vi "Read presence_penalty.vi"(8 "error in (no error)":errorcluster, 11 "abstract_llm_base in":refnum<class "abstract_llm_base.lvclass">) -> (0 "error out":errorcluster, 2 "presence_penalty":dbl, 3 "abstract_llm_base out":refnum<class "abstract_llm_base.lvclass">)   [LabVIEW 2020, in "abstract_llm_base.lvclass"]
uses:
  abstract_llm_base.lvclass
  abstract_llm_base.lvclass/abstract_llm_base.ctl
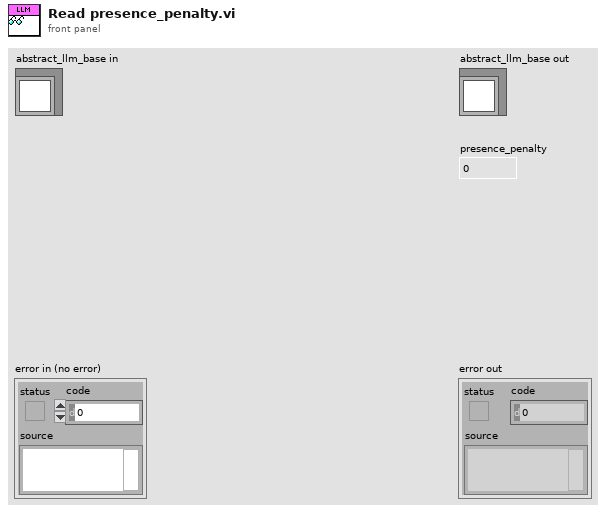
[diagram p1: front panel]
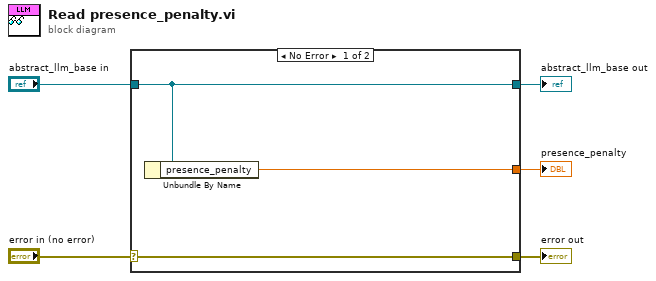
[diagram p0: block diagram]
diagram:
  n1 = case shown="No Error" "error in (no error)" {
    selector: "error in (no error)" -> [w8 w9]
    tunnel: [w8 w9] -> w4
    tunnel: [w7 w10] -> w2
    tunnel: "abstract_llm_base in" -> [w7 w10]
    tunnel: [w6 _] -> w1
    frame No Error {
      n2 = Unbundle By Name(w7) -> ("presence_penalty"=w6:dbl)
    }
    frame Error {
    }
  }
  "error out" <- w4
  "abstract_llm_base out" <- w2
  "presence_penalty" <- w1
